vi "Interpolate 2D main.vi"(4 "ntimes":i32=1, 6 "yi":dbl[][](array[numeric]), 7 "method":i32(ring)=1 items=["nearest", "bilinear", "bicubic", "bicubic spline"], 8 "xi":dbl[][](array[numeric]), 9 "Y":dbl[][](array[numeric]), 10 "X":dbl[][](array[numeric]), 11 "Z":dbl[][](array[numeric])) -> (0 "error":i32, 1 "yi used":dbl[][](array[numeric]), 2 "xi used":dbl[][](array[numeric]), 3 "zi":dbl[][](array[numeric]))   [LabVIEW 2013, in "NI_Gmath.lvlib"]
uses:
  NI_Gmath.lvlib
panel:
  # "Interpolate 2D"
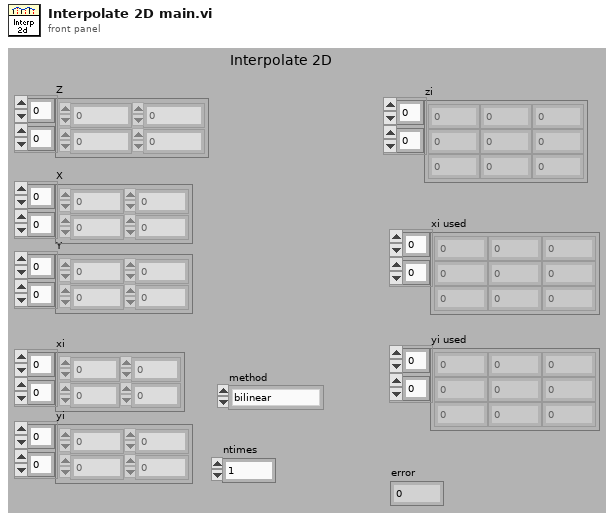
[diagram p1: front panel]
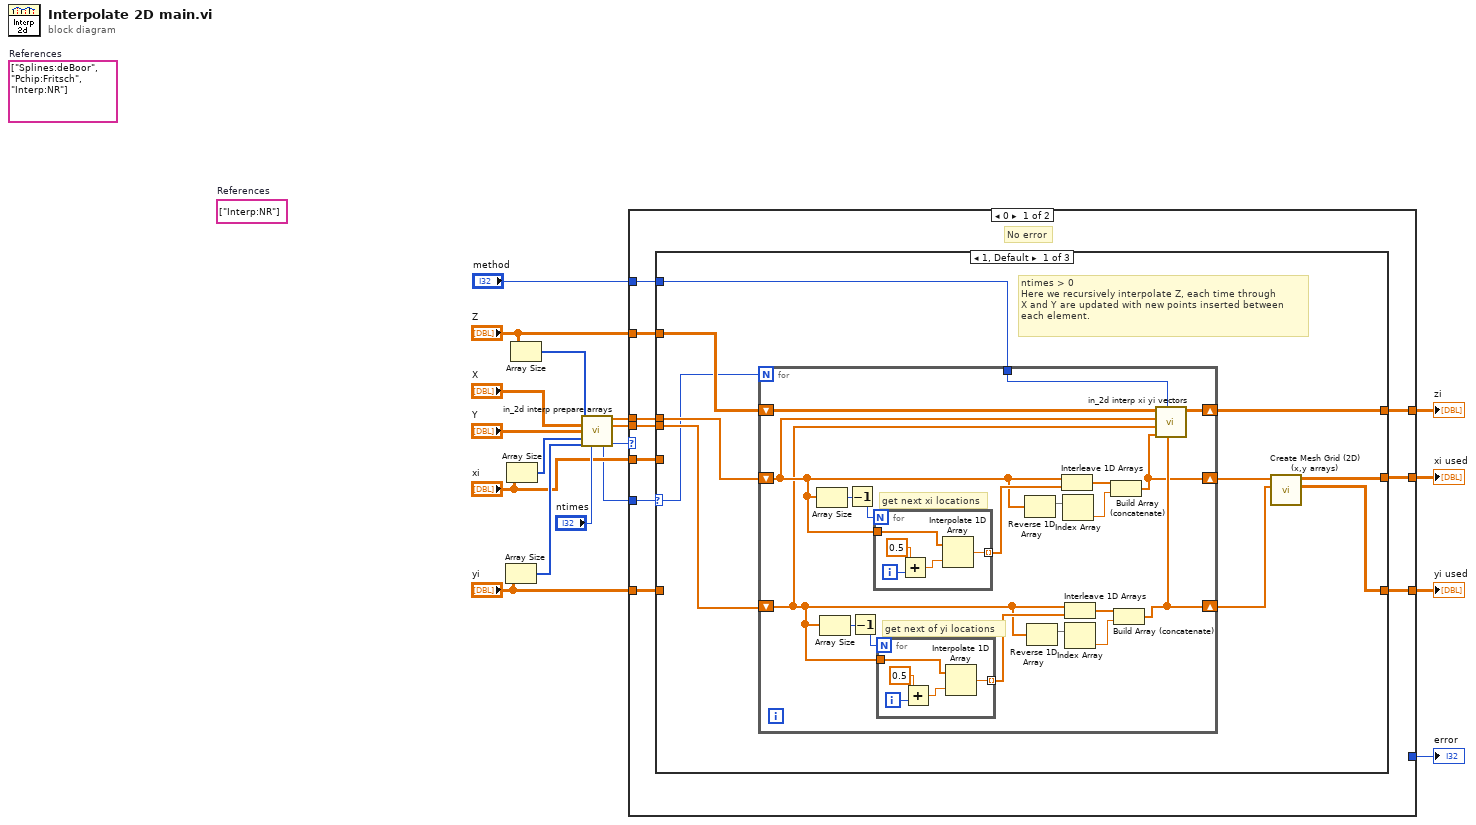
[diagram p0: block diagram]
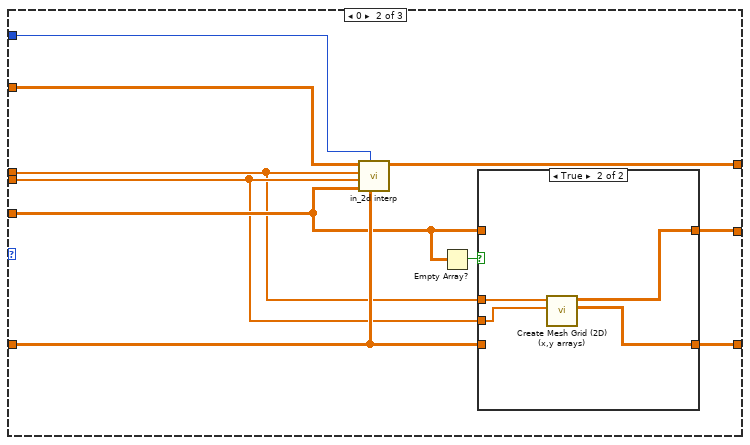
[diagram p2: hidden frame]
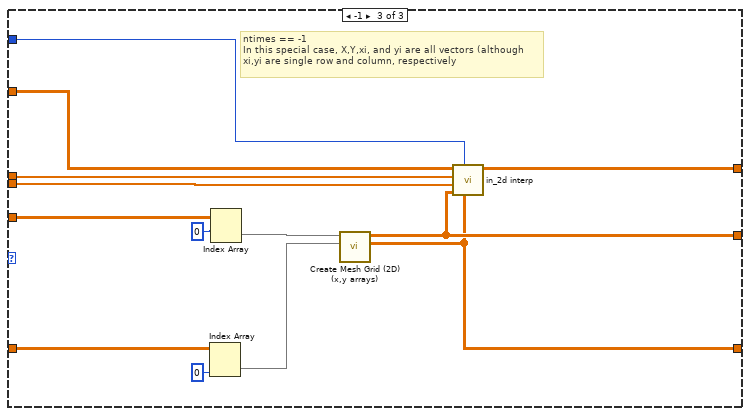
[diagram p4: hidden frame]
diagram:
  (unwired) string[] ["Interp:NR"]  # References
  (unwired) string[] ["Splines:deBoor", "Pchip:Fritsch", "Interp:NR"]  # References
  n1 = Array Size(array="yi") -> (size(s)=w7:i32[])
  n2 = Array Size(array="xi") -> (size(s)=w6:i32[])
  n3 = Array Size(array="Z") -> (size(s)=w17:i32[])
  n4 = call "in_2d interp prepare arrays.vi"("size of Z"=w17, "X"="X", "Y"="Y", "xi size"=w6, "yi size"=w7, "ntimes"="ntimes") -> ("X-out"=w12:dbl[], "Y-out"=w4:dbl[], "ntimes remaining"=w1:i32, "error"=w3:i32)  [unwired: 5 in, 1 out]
  n5 = case shown="0" w3 {
    selector: w3 -> [_ w97]
    tunnel: [w28 _] -> w14
    tunnel: "Z" -> [w27 _]
    tunnel: w12 -> [w26 _]
    tunnel: "method" -> [w25 _]
    tunnel: [w24 _] -> w10
    tunnel: [w23 _] -> w9
    tunnel: "yi" -> [w22 _]
    tunnel: "xi" -> [w21 _]
    tunnel: w1 -> [w20 _]
    tunnel: w4 -> [w19 _]
    tunnel: [_ w97] -> w2
    frame 0 {
      # "No error"
      n6 = case shown="1, Default" w20 {
        selector: w20 -> [w33 _ _]
        tunnel: [w38 w77 w85] -> w28
        tunnel: w27 -> [w37 w76 w90]
        tunnel: w26 -> [w35 w68 w89]
        tunnel: w19 -> [w34 w69 w88]
        tunnel: w21 -> [_ w70 w96]
        tunnel: w22 -> [_ w72 w94]
        tunnel: w25 -> [w36 w75 w87]
        tunnel: [w29 w71 w84] -> w24
        tunnel: [w30 w73 w86] -> w23
        frame 1, Default {
          # "ntimes > 0\nHere we recursively interpolate Z, each time through\nX and Y are updated with new points inserted between\neach element."
          n7 = for {
            N: w33 -> [_]
            tunnel: w36 -> [w55]
            shift-right: [w42] -> w31
            shift-left: w34 -> [w39]
            shift-right: [w57] -> w38
            shift-left: w37 -> [w56]
            shift-right: [w41] -> w32
            shift-left: w35 -> [w40]
            # "get next of yi locations"
            # "get next xi locations"
            n8 = Array Size(array=w40) -> (size(s)=w54:i32)
            n9 = Array Size(array=w39) -> (size(s)=w48:i32)
            n10 = Decrement(x=w54) -> (x-1=w53:i32)
            n11 = Decrement(x=w48) -> (x-1=w47:i32)
            n12 = for {
              N: w53 -> [_]
              tunnel: [w67] -> w51 mode=indexing
              tunnel: w40 -> [w63]
              i -> [w65]
              n13 = Add(x=0.5, y=w65) -> (x+y=w64:dbl)
              n14 = Interpolate 1D Array(1:w64, 2:w63) -> (0:w67:dbl)
            }
            n15 = for {
              N: w47 -> [_]
              tunnel: [w62] -> w43 mode=indexing
              tunnel: w39 -> [w58]
              i -> [w60]
              n16 = Add(x=0.5, y=w60) -> (x+y=w59:dbl)
              n17 = Interpolate 1D Array(1:w59, 2:w58) -> (0:w62:dbl)
            }
            n18 = Reverse 1D Array(array=w40) -> (reversed array=w52:dbl[])
            n19 = Reverse 1D Array(array=w39) -> (reversed array=w46:dbl[])
            n20 = Interleave 1D Arrays(w40, w51) -> (w49:dbl[])
            n21 = Index Array(array=w52) -> (element=w50:dbl)  [unwired: 1 in]
            n22 = Interleave 1D Arrays(w39, w43) -> (w44:dbl[])
            n23 = Index Array(array=w46) -> (element=w45:dbl)  [unwired: 1 in]
            n24 = Build Array (concatenate)(w49, w50) -> (w41:dbl[])
            n25 = Build Array (concatenate)(w44, w45) -> (w42:dbl[])
            n26 = call "in_2d interp xi yi vectors.vi"("yi"=w42, "method"=w55, "xi"=w41, "Y"=w39, "X"=w40, "Z"=w56) -> ("zi"=w57:dbl[][])  [unwired: 5 in]
          }
          n27 = call "Create Mesh Grid (2D) (x,y arrays).vi"("y domain"=w31, "x domain"=w32) -> ("Y"=w29:dbl[][], "X"=w30:dbl[][])  [unwired: 7 in, 1 out]
        }
        frame 0 {
          n28 = call "in_2d interp.vi"("yi"=w72, "method"=w75, "xi"=w70, "Y"=w69, "X"=w68, "Z"=w76) -> ("zi"=w77:dbl[][])  [unwired: 5 in]
          n29 = Empty Array?(array=w70) -> (empty?=w74:bool)
          n30 = case shown="True" w74 {
            tunnel: w70 -> [w79 _]
            tunnel: [w79 w81] -> w73
            tunnel: w72 -> [w78 _]
            tunnel: [w78 w80] -> w71
            tunnel: w69 -> [_ w82]
            tunnel: w68 -> [_ w83]
            frame False {
            }
            frame True {
              n31 = call "Create Mesh Grid (2D) (x,y arrays).vi"("y domain"=w82, "x domain"=w83) -> ("Y"=w80:dbl[][], "X"=w81:dbl[][])  [unwired: 7 in, 1 out]
            }
          }
        }
        frame -1 {
          # "ntimes == -1\nIn this special case, X,Y,xi, and yi are all vectors (although\nxi,yi are single row and column, respectively"
          n32 = Index Array(array=w94, index (col)=0 ("index (row)")) -> (element=w91:dbl[])  [unwired: 1 in]
          n33 = Index Array(array=w96, index (row)=0) -> (element=w92:dbl[])  [unwired: 1 in]
          n34 = call "Create Mesh Grid (2D) (x,y arrays).vi"("y domain"=w91, "x domain"=w92) -> ("Y"=w84:dbl[][], "X"=w86:dbl[][])  [unwired: 7 in, 1 out]
          n35 = call "in_2d interp.vi"("yi"=w84, "method"=w87, "xi"=w86, "Y"=w88, "X"=w89, "Z"=w90) -> ("zi"=w85:dbl[][])  [unwired: 5 in]
        }
      }
    }
    frame 1, Default {
      # "Error"
    }
  }
  "zi" <- w14
  "xi used" <- w9
  "yi used" <- w10
  "error" <- w2
